vi "setGPGFolder.vi"(0 "HGF_GPG":refnum<class "HGF_GPG.lvclass">, 2 "gpg working directory":path, 5 "error in (no error)":errorcluster) -> (14 "dup HGF_GPG":refnum<class "HGF_GPG.lvclass">, 19 "error out":errorcluster)   [LabVIEW 2012, in "HGF_GPG.lvlib" / "HGF_GPG.lvclass"]
doc: "Set the GPG working folder. Must be set for the GPG functions will work correctly"
uses:
  HGF_GPG.lvclass
  HGF_GPG.lvclass/HGF_GPG.ctl
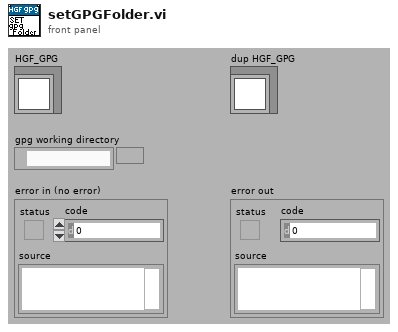
[diagram p1: front panel]
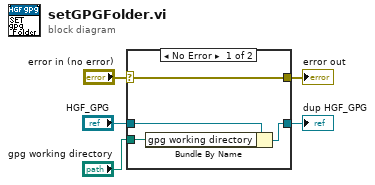
[diagram p0: block diagram]
diagram:
  n1 = case shown="No Error" "error in (no error)" {
    selector: "error in (no error)" -> [w8 w11]
    tunnel: "HGF_GPG" -> [w9 w10]
    tunnel: [w7 w10] -> w4
    tunnel: [w8 w11] -> w2
    tunnel: "gpg working directory" -> [w6 _]
    frame No Error {
      n2 = Bundle By Name(cluster=w9, "gpg working directory"=w6) -> (w7:refnum<class "HGF_GPG.lvclass">)
    }
    frame Error {
    }
  }
  "dup HGF_GPG" <- w4
  "error out" <- w2
